vi "Read Order Total Cost.vi"(8 "error in (no error)":errorcluster, 11 "Order in":refnum<class "Order.lvclass">) -> (0 "error out":errorcluster, 2 "Order Total Cost":dbl, 3 "Order out":refnum<class "Order.lvclass">)   [LabVIEW 2020, in "Order.lvclass"]
uses:
  Order.lvclass
  Order.lvclass/Order.ctl
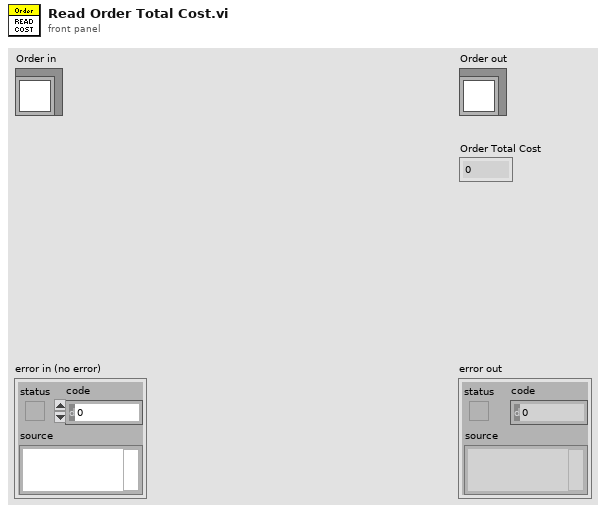
[diagram p1: front panel]
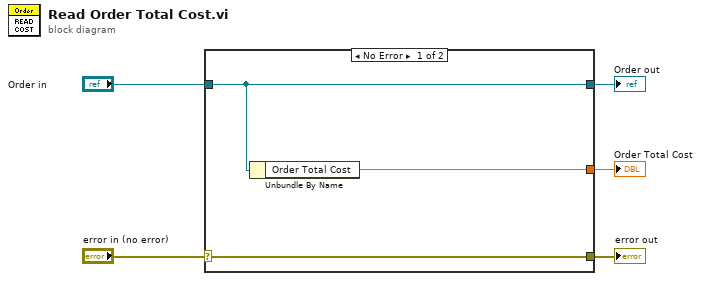
[diagram p0: block diagram]
diagram:
  n1 = case shown="No Error" "error in (no error)" {
    selector: "error in (no error)" -> [w8 w9]
    tunnel: [w8 w9] -> w4
    tunnel: [w7 w10] -> w2
    tunnel: "Order in" -> [w7 w10]
    tunnel: [w6 _] -> w1
    frame No Error {
      n2 = Unbundle By Name(w7) -> ("Order Total Cost"=w6:dbl)
    }
    frame Error {
    }
  }
  "error out" <- w4
  "Order out" <- w2
  "Order Total Cost" <- w1
